vi "ex1.vi"() -> ()   [LabVIEW 2022 SP3]
uses:
  #typedef_ex1_states.ctl
panel:
  out "Result":string
  in  "Calculator":T1
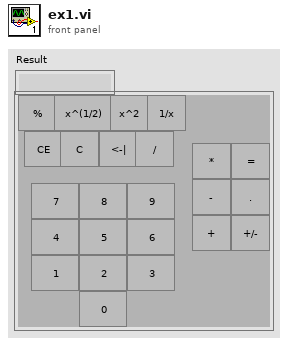
[diagram p1: front panel]
types:
  T1 = cluster{"Press 0":bool, "Press 1":bool, "Press 2":bool, "Press 3":bool, "Press 4":bool, "Press 5":bool, "Press 6":bool, "Press 7":bool, "Press 8":bool, "Press 9":bool, "Multiple":bool, "Substraction":bool, "Adding":bool, "Equal":bool, "Period":bool, "Change Sign":bool, "Percentage":bool, "Square Root":bool, "Square":bool, "1/x":bool, "CE":bool, "C":bool, "Delete":bool, "Divide":bool}
  T2 = typedef "#typedef_ex1_states.ctl" = enum16{"period", "sign change", "mul", "1/x", "del", "per", "c", "ce", "sqr", "sq", "sub", "div", "add", "Error Handler", "Exit", "Initialize", "WaitForEvent", "OpartionWasDone"}
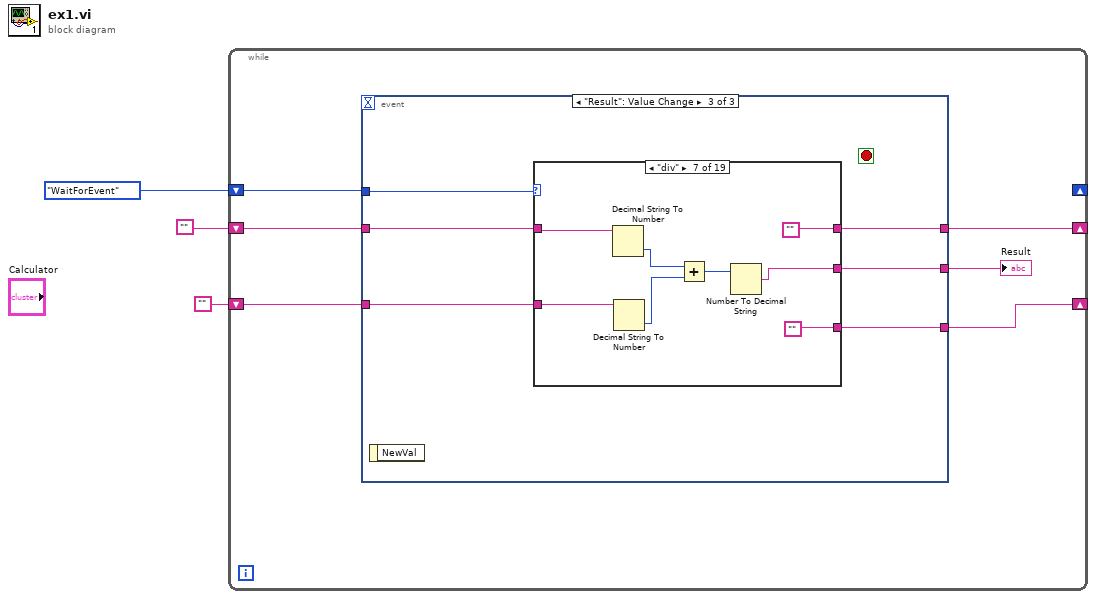
[diagram p0: block diagram]
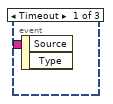
[diagram p2: hidden frame]
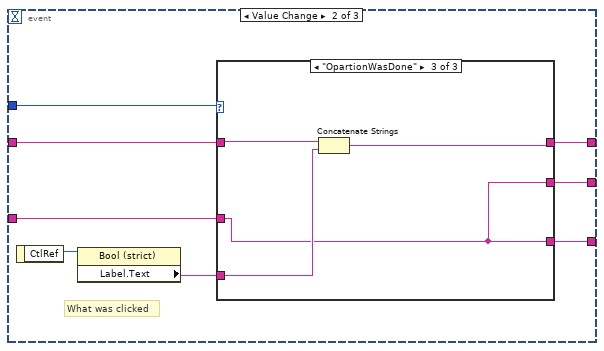
[diagram p3: hidden frame]
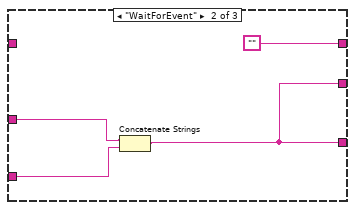
[diagram p5: hidden frame]
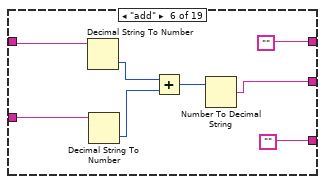
[diagram p11: hidden frame]
diagram:
  n1 = while {
    shift-right: _ -> [_]
    shift-left: #typedef_ex1_states."WaitForEvent" ("Enum") -> [w9]
    shift-right: [w5] -> _
    shift-left: "" -> [w8]
    shift-right: [w6] -> _
    shift-left: "" -> [w7]
    stop <- _ stop-if-true
    n2 = event shown="[2] \"Result\": Value Change" {
      selector: _ -> [_ _ _]
      dyn-events: _ -> [_ _ _]
      timeout: _ -> [_ _ _]
      tunnel: w9 -> [_ w16 w31]
      tunnel: w8 -> [_ w15 w30]
      tunnel: w7 -> [_ w13 w29]
      tunnel: [_ w12 w28] -> w6
      tunnel: [_ w11 w26] -> w5
      tunnel: [_ w10 w27] -> w4
      event Timeout {
        n3 = event-data() -> ()  [unwired: 1 in, 2 out]
      }
      event "Calculator.Press 0", "Calculator.Press 1", "Calculator.Press 2", "Calculator.Press 3", "Calculator.Press 4", "Calculator.Press 5", "Calculator.Press 6", "Calculator.Press 7", "Calculator.Press 8", "Calculator.Press 9": Value Change {
        # "What was clicked"
        n4 = event-data() -> ("CtlRef"=w17:refnum<vi>)  [unwired: 1 in]
        n5 = property class="Bool (strict)"(reference=w17) -> ("Label.Text"=w14:string)  [unwired: 1 in, 2 out]
        n6 = case shown="\"OpartionWasDone\"" w16 {
          tunnel: w15 -> [_ _ w25]
          tunnel: w14 -> [_ w21 w24]
          tunnel: w13 -> [_ w20 w22]
          tunnel: [_ w18 w22] -> w12
          tunnel: [_ "" w23] -> w11
          tunnel: [_ w18 w22] -> w10
          frame "Error Handler", Default {
          }
          frame "WaitForEvent" {
            n7 = Concatenate Strings(w20, w21) -> (w18:string)
          }
          frame "OpartionWasDone" {
            n8 = Concatenate Strings(w25, w24) -> (w23:string)
          }
        }
      }
      event "Result": Value Change {
        n9 = event-data() -> ()  [unwired: 1 in, 1 out]
        n10 = case shown="\"div\"" w31 {
          tunnel: w30 -> [_ w32 _ _ _ w41 w49 _ _ _ _ _ _ _ _ _ _ _ _]
          tunnel: w29 -> [_ w33 _ _ _ w39 w47 _ _ _ _ _ _ _ _ _ _ _ _]
          tunnel: [_ w33 _ _ _ "" "" _ _ _ _ _ _ _ _ _ _ _ _] -> w28
          tunnel: [_ w33 _ _ _ w36 w44 _ _ _ _ _ _ _ _ _ _ _ _] -> w27
          tunnel: [_ w32 _ _ _ "" "" _ _ _ _ _ _ _ _ _ _ _ _] -> w26
          frame "Error Handler", Default {
          }
          frame "WaitForEvent" {
          }
          frame "OpartionWasDone" {
          }
          frame "Exit" {
          }
          frame "Initialize" {
          }
          frame "add" {
            n11 = Decimal String To Number(string=w41) -> (number=w40:i32)  [unwired: 2 in, 1 out]
            n12 = Decimal String To Number(string=w39) -> (number=w38:i32)  [unwired: 2 in, 1 out]
            n13 = Add(x=w40, y=w38) -> (x+y=w37:i32)
            n14 = Number To Decimal String(number=w37) -> (decimal integer string=w36:string)  [unwired: 1 in]
          }
          frame "div" {
            n15 = Decimal String To Number(string=w49) -> (number=w48:i32)  [unwired: 2 in, 1 out]
            n16 = Decimal String To Number(string=w47) -> (number=w46:i32)  [unwired: 2 in, 1 out]
            n17 = Add(x=w48, y=w46) -> (x+y=w45:i32)
            n18 = Number To Decimal String(number=w45) -> (decimal integer string=w44:string)  [unwired: 1 in]
          }
          frame "div" {
          }
          frame "sub" {
          }
          frame "sq" {
          }
          frame "sqr" {
          }
          frame "ce" {
          }
          frame "c" {
          }
          frame "per" {
          }
          frame "del" {
          }
          frame "1/x" {
          }
          frame "mul" {
          }
          frame "sign change" {
          }
          frame "period" {
          }
        }
      }
    }
    "Result" <- w4
  }
